vi "LT_init_two.vi"(0 "VISA1":refnum<vi>, 3 "VISA2":refnum<vi>, 5 "error in":errorcluster, 8 "SN":string[](array[string])=["240804202", "240804204"]) -> (14 "VISA1 out":refnum<visa-resource-name>, 15 "dev_param_1":T1={"Length of data block"=14, "Converter address"=0, "Converter type"=180, "PZD1"=0, "PZD2"=0} {"Converter type" items=["Turbovac 350/450 i"=180, "Turbovac 350/450 i with optional interface"=181, "Turbovac 350/450 iX"=182, "Turbovac  90/250 i"=190, "Turbovac  90/250 with optional interface"=191, "Turbovac  90/250 iX"=192, "Turbovac  850/950 i"=195, "Turbovac  850/950 i with optional interface"=196, "Turbovac  850/950 iX"=197, "Turbovac 1350/1450 i"=185, "Turbovac 1350/1450 i with optional interface"=186, "Turbovac 1350/1450 iX"=187]; "Length of data block" items=["14"=14, "22"=22]}, 16 "error1":errorcluster, 17 "VISA2 out":refnum<visa-resource-name>, 18 "dev_param_2":T1={"Length of data block"=14, "Converter address"=0, "Converter type"=180, "PZD1"=0, "PZD2"=0} {"Converter type" items=["Turbovac 350/450 i"=180, "Turbovac 350/450 i with optional interface"=181, "Turbovac 350/450 iX"=182, "Turbovac  90/250 i"=190, "Turbovac  90/250 with optional interface"=191, "Turbovac  90/250 iX"=192, "Turbovac  850/950 i"=195, "Turbovac  850/950 i with optional interface"=196, "Turbovac  850/950 iX"=197, "Turbovac 1350/1450 i"=185, "Turbovac 1350/1450 i with optional interface"=186, "Turbovac 1350/1450 iX"=187]; "Length of data block" items=["14"=14, "22"=22]}, 19 "error2":errorcluster)   [LabVIEW 2019]
uses:
  <instrlib>/Leybold TURBOVAC/Public/Ctl/Device Parameters Indicator.ctl
  <instrlib>/Leybold TURBOVAC/Public/Ctl/Converter Type Indicator.ctl
  <vilib>/Utility/error.llb/Error Cluster From Error Code.vi
  <vilib>/ErrorRing/Error Ring.xnode
  <instrlib>/Leybold TURBOVAC/Leybold TURBOVAC.lvlib
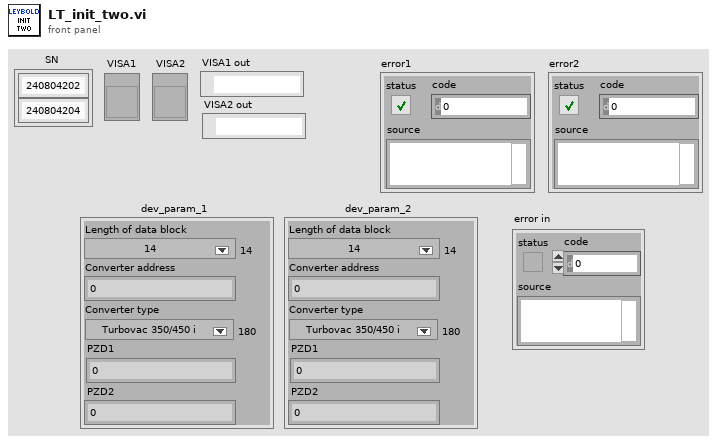
[diagram p1: front panel]
types:
  T1 = typedef "Leybold TURBOVAC.lvlib/Device Parameters Indicator.ctl" = cluster{"Length of data block":u8, "Converter address":u8, "Converter type":T2, "PZD1":u16, "PZD2":u16}
  T2 = typedef "Leybold TURBOVAC.lvlib/Converter Type Indicator.ctl" = u16
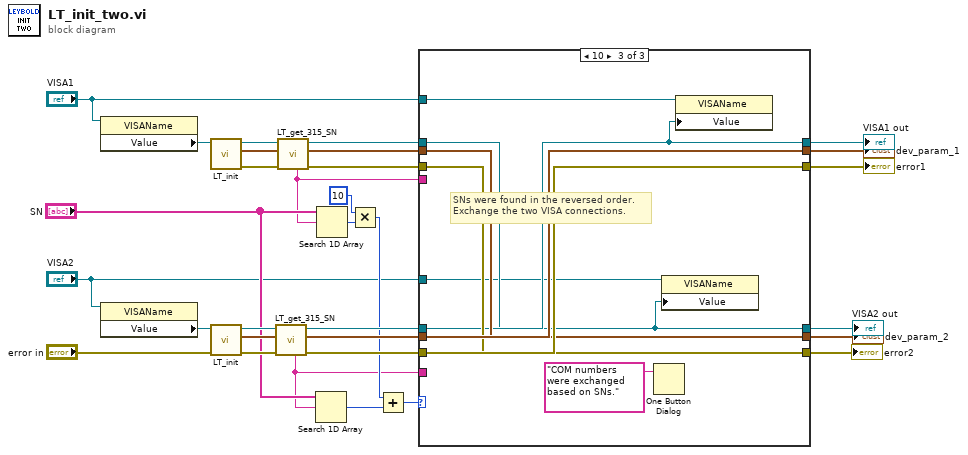
[diagram p0: block diagram]
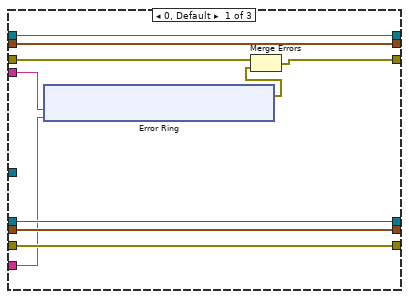
[diagram p2: hidden frame]
diagram:
  n1 = property on="Property Node" class="VISAName"(reference="VISA1") -> ("Value"=w11:refnum<visa-resource-name>)  [unwired: 1 in, 2 out]
  n2 = property on="Property Node" class="VISAName"(reference="VISA2") -> ("Value"=w9:refnum<visa-resource-name>)  [unwired: 1 in, 2 out]
  n3 = call "LT_init.vi"("VISA in"=w11) -> ("error out"=w29:errorcluster, "dev_param_out"=w30:T1, "VISA out"=w31:refnum<visa-resource-name>)  [unwired: 7 in, 1 out]
  n4 = call "LT_init.vi"("error in"="error in", "VISA in"=w9) -> ("error out"=w26:errorcluster, "dev_param_out"=w27:T1, "VISA out"=w28:refnum<visa-resource-name>)  [unwired: 6 in, 1 out]
  n5 = call "LT_get_315_SN.vi"("error in"=w26, "dev_param_in"=w27, "VISA in"=w28) -> ("error out"=w20:errorcluster, "dev_param_out"=w21:T1, "VISA out"=w22:refnum<visa-resource-name>, "SN_converter"=w12:string)  [unwired: 5 in]
  n6 = call "LT_get_315_SN.vi"("error in"=w29, "dev_param_in"=w30, "VISA in"=w31) -> ("error out"=w23:errorcluster, "dev_param_out"=w24:T1, "VISA out"=w25:refnum<visa-resource-name>, "SN_converter"=w13:string)  [unwired: 5 in]
  n7 = Search 1D Array(1D array="SN", element=w12) -> (index of element=w15:i32)  [unwired: 1 in]
  n8 = Search 1D Array(1D array="SN", element=w13) -> (index of element=w18:i32)  [unwired: 1 in]
  n9 = Multiply(x=10, y=w18) -> (x*y=w16:i32)
  n10 = Add(x=w16, y=w15) -> (x+y=w14:i32)
  n11 = case shown="10" w14 {
    tunnel: w25 -> [w41 w51 w57]
    tunnel: w24 -> [w40 w54 w62]
    tunnel: w23 -> [w36 w55 w61]
    tunnel: [w35 w55 w64] -> w5
    tunnel: [w40 w54 w63] -> w3
    tunnel: [w41 w51 w58] -> w7
    tunnel: w22 -> [w39 w50 w58]
    tunnel: w21 -> [w38 w53 w63]
    tunnel: w20 -> [w37 w52 w64]
    tunnel: [w39 w50 w57] -> w6
    tunnel: [w38 w53 w62] -> w2
    tunnel: [w37 w52 w61] -> w4
    tunnel: w13 -> [w33 _ _]
    tunnel: w12 -> [w32 _ _]
    tunnel: "VISA1" -> [_ _ w59]
    tunnel: "VISA2" -> [_ _ w56]
    frame 0, Default {
      n12 = xnode "Error Ring"("parameter 0"=w33, "parameter 1"=w32) -> ("error out"=w34:errorcluster)
      n13 = Merge Errors(w36, w34) -> (w35:errorcluster)
    }
    frame 1 {
      # "SNs were found in the normal order."
    }
    frame 10 {
      # "SNs were found in the reversed order.\nExchange the two VISA connections."
      n14 = One Button Dialog(message="COM numbers were exchanged based on SNs.") -> ()  [unwired: 1 in, 1 out]
      n15 = property class="VISAName"(reference=w56, "Value"=w57) -> ()  [unwired: 1 in, 2 out]
      n16 = property class="VISAName"(reference=w59, "Value"=w58) -> ()  [unwired: 1 in, 2 out]
    }
  }
  "VISA1 out" <- w7
  "VISA2 out" <- w6
  "error1" <- w5
  "error2" <- w4
  "dev_param_1" <- w3
  "dev_param_2" <- w2
